vi "Write (I64).vi"(9 "error in (no error)":errorcluster, 10 "I64 Value":i64, 11 "Config Element in":refnum<class "Config Element.lvclass">) -> (1 "error out":errorcluster, 3 "Config Element out":refnum<class "Config Element.lvclass">)   [LabVIEW 2020, in "CDM-Config.lvlib" / "Config Element.lvclass"]
uses:
  Config Element.lvclass
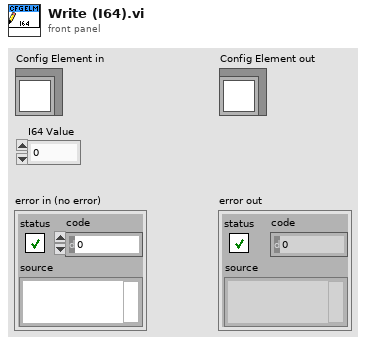
[diagram p1: front panel]
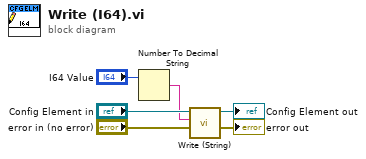
[diagram p0: block diagram]
diagram:
  n1 = Number To Decimal String(number="I64 Value") -> (decimal integer string=w1:string)  [unwired: 1 in]
  n2 = call "Write (String).vi"("error in (no error)"="error in (no error)", "String Value"=w1, "Config Element in"="Config Element in") -> ("error out"=→"error out":errorcluster, "Config Element out"=→"Config Element out":refnum<class "Config Element.lvclass">)  [unwired: 7 in]
